vi "FTW-Test-Reflection-Datatypes.vi"() -> (0 "Test Result":errorcluster)   [LabVIEW 2014]
uses:
  src/reflection/FTW-Reflection-Types.ctl
  src/database/core/FTW-SQLite-Core-AccessMode.ctl
  src/socket/inbox/core/FTW-Inbox-Core-Type.ctl
  src/json/core/FTW-JSON-Core-Structure.ctl
  src/error/FTW-ERR-ThrowError.vi
  src/error/FTW-ERR-CallChain.vi
  src/string/FTW-STR-ReplaceWhitespace.vi
panel:
  out "Results Array":T2(array[cluster])
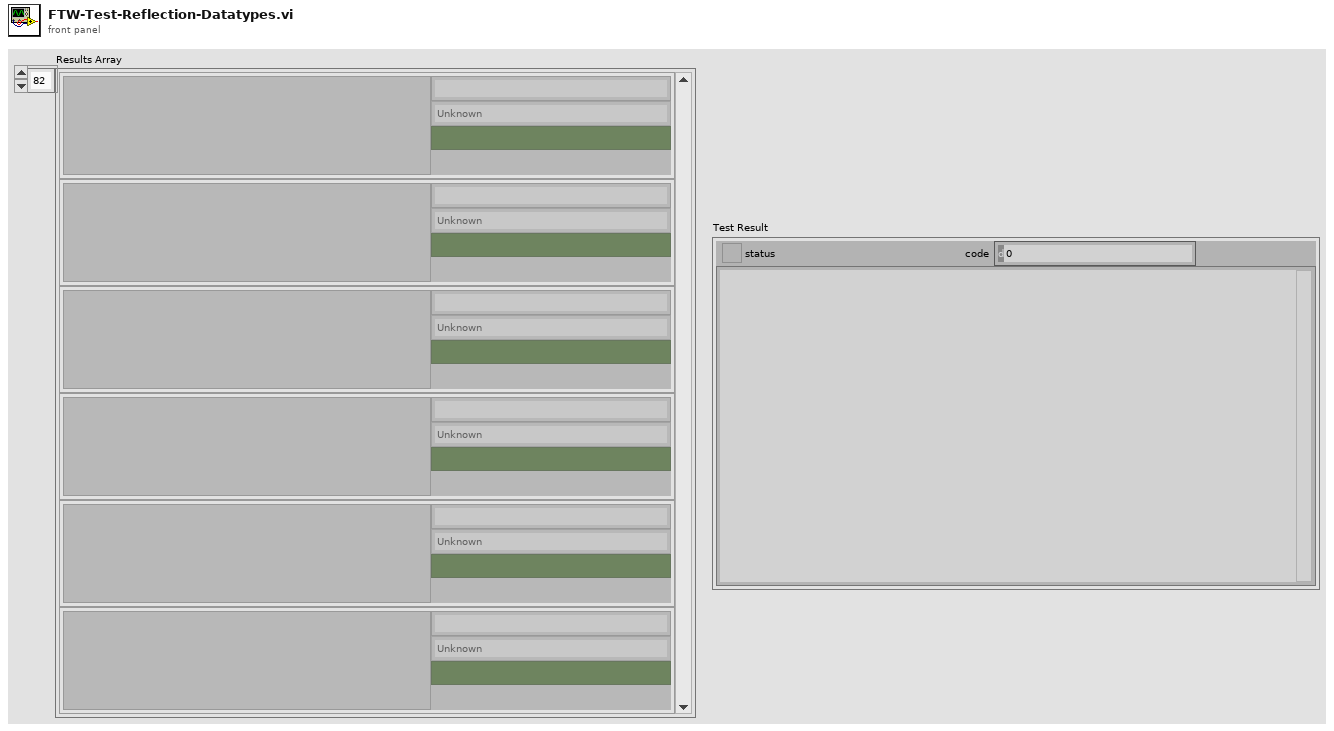
[diagram p1: front panel]
types:
  T1 = typedef "FTW-Reflection-Types.ctl" = enum16{"Unknown", "Void", "Array", "Cluster", "LVObject", "Boolean", "I8", "I16", "I32", "I64", "U8", "U16", "U32", "U64", "SGL", "DBL", "EXT", "CSG", "CDB", "CXT", "FXP", "EnumU8", "EnumU16", "EnumU32", "EnumU64", "SGLwithUnit", "DBLwithUnit", "EXTwithUnit", "CSGwithUnit", "CDBwithUnit", "CXTwithUnit", "String", "Path", "Picture", "Tag", "LVVariant", "Timestamp", "WaveformI8", "WaveformI16", "WaveformI32", "WaveformI64", "WaveformU8", "WaveformU16", "WaveformU32", "WaveformU64", "WaveformSGL", "WaveformDBL", "WaveformEXT", "WaveformCSG", "WaveformCDB", "WaveformCXT", "WaveformDigital", "WaveformUnknownType", "DigitalData", "DynamicData", "ExternalData", "FileByteStream", "TDMStream", "dotNET", "ActiveX", "VIServerReference", "VIReference", "ApplicationInstance", "Menu", "ConnectionDataSocket", "ConnectionVISA", "ConnectionBluetooth", "ConnectionIrDA", "ConnectionTCP", "ConnectionUDP", "ConnectionHTTPClient", "ConnectionFTP", "Occurrence", "Notifier", "Queue", "Rendezvous", "Semaphore", "RTFIFO", "EventPublisher", "EventRegistration", "EventCallback", "DataValueReference", "GenericClass", "GenericClassTag", "GenericClassDeepCopy", "GenericClassFlattened", "GenericClassTagFlattened", "GenericReferenceType", "WindowsRegistry", "OverloadedDatalogRef", "ReferenceUnknownType", "ByteArray", "ConPaneInterface"}
  T2 = cluster{"Variant":variant, "xml string":string, "LabVIEW Type":T1, "Pass?":bool}[]
  T3 = typedef "FTW-Inbox-Core-Type.ctl" = cluster{"Socket":i64, "MessageNotifier":refnum<user-event>, "Message Broker":refnum<user-event>}
  T4 = typedef "Rendezvous RefNum" = refnum<k1>
  T5 = typedef "Semaphore RefNum" = refnum<k1>
  T6 = typedef "FTW-SQLite-Core-AccessMode.ctl" = enum16{"Read", "Read/Write", "Read/Write/Create"}
  T7 = cluster{"Variant":variant, "Match":string, "LabVIEW Type":T1, "Status OK?":bool}
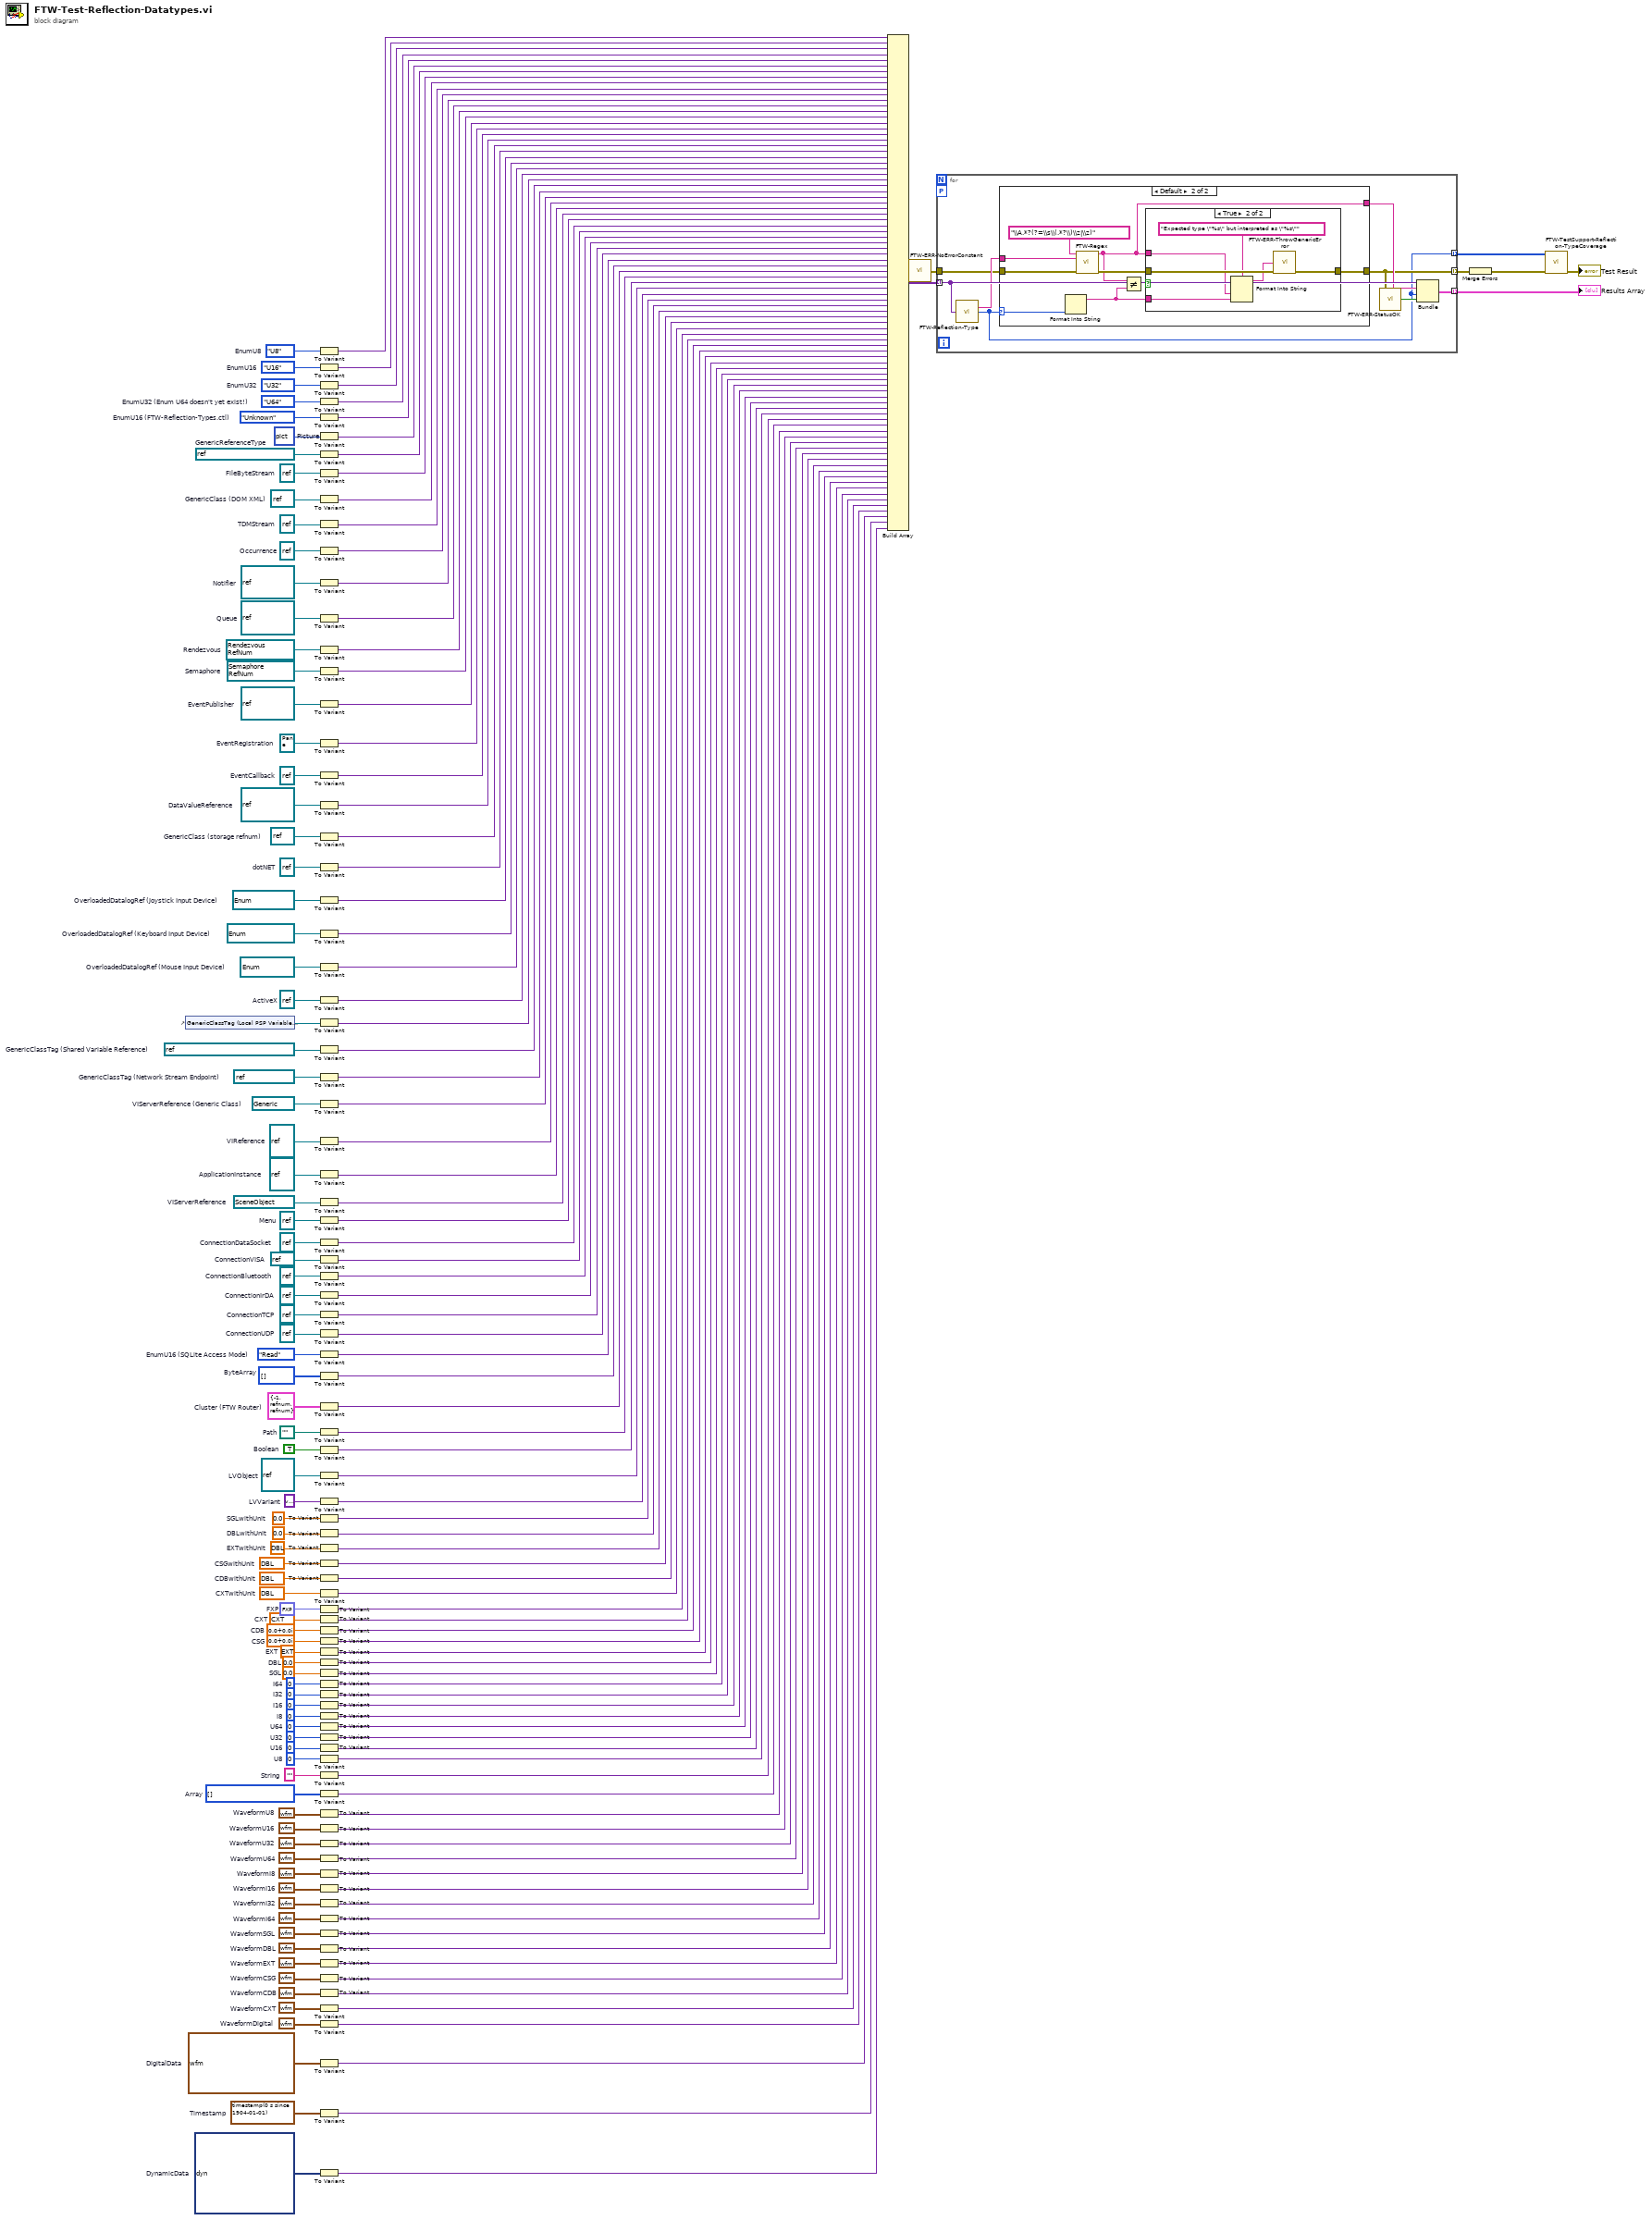
[diagram p0: block diagram]
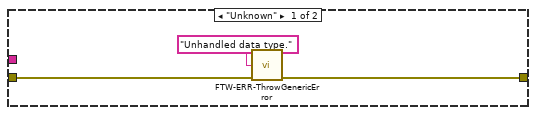
[diagram p2: hidden frame]
diagram:
  w21 = dynamicdata []  # DynamicData
  w5 = u8[] []  # ByteArray
  w6 = T3 {"Socket"=-1, "MessageNotifier"=refnum, "Message Broker"=refnum}  # Cluster (FTW Router)
  w14 = u16[] []  # Array
  w13 = ""  # String
  w9 = T4 refnum items=["rendezvous"]  # Rendezvous
  w8 = T5 refnum items=["semaphore"]  # Semaphore
  w17 = enum32{"U64"}."U64"  # EnumU32 (Enum U64 doesn't yet exist!)
  w20 = FTW-SQLite-Core-AccessMode."Read"  # EnumU16 (SQLite Access Mode)
  w23 = digitalwaveform {"t0"=timestamp(0 s since 1904-01-01), "dt"=0.0, "Y"={"transitions"=[], "data"=[]}}  # WaveformDigital
  w24 = waveform(cxt) {"t0"=timestamp(0 s since 1904-01-01), "dt"=1.0, "Y"=[]}  # WaveformCXT
  w25 = waveform(cdb) {"t0"=timestamp(0 s since 1904-01-01), "dt"=1.0, "Y"=[]}  # WaveformCDB
  w26 = waveform(csg) {"t0"=timestamp(0 s since 1904-01-01), "dt"=1.0, "Y"=[]}  # WaveformCSG
  w27 = waveform(ext) {"t0"=timestamp(0 s since 1904-01-01), "dt"=1.0, "Y"=[]}  # WaveformEXT
  w28 = waveform(dbl) {"t0"=timestamp(0 s since 1904-01-01), "dt"=1.0, "Y"=[]}  # WaveformDBL
  w29 = waveform(sgl) {"t0"=timestamp(0 s since 1904-01-01), "dt"=1.0, "Y"=[]}  # WaveformSGL
  w30 = waveform(i64) {"t0"=timestamp(0 s since 1904-01-01), "dt"=1.0, "Y"=[]}  # WaveformI64
  w31 = waveform(i32) {"t0"=timestamp(0 s since 1904-01-01), "dt"=1.0, "Y"=[]}  # WaveformI32
  w32 = waveform(i16) {"t0"=timestamp(0 s since 1904-01-01), "dt"=1.0, "Y"=[]}  # WaveformI16
  w36 = waveform(i8) {"t0"=timestamp(0 s since 1904-01-01), "dt"=1.0, "Y"=[]}  # WaveformI8
  w37 = waveform(u64) {"t0"=timestamp(0 s since 1904-01-01), "dt"=1.0, "Y"=[]}  # WaveformU64
  w35 = waveform(u32) {"t0"=timestamp(0 s since 1904-01-01), "dt"=1.0, "Y"=[]}  # WaveformU32
  w34 = waveform(u16) {"t0"=timestamp(0 s since 1904-01-01), "dt"=1.0, "Y"=[]}  # WaveformU16
  w33 = waveform(u8) {"t0"=timestamp(0 s since 1904-01-01), "dt"=1.0, "Y"=[]}  # WaveformU8
  w110 = refnum<k31> refnum  # ConnectionBluetooth
  w81 = enum32{"U32"}."U32"  # EnumU32
  w80 = enum16{"U16"}."U16"  # EnumU16
  w79 = enum8{"U8"}."U8"  # EnumU8
  w114 = TRUE  # Boolean
  w115 = path ""  # Path
  w82 = FTW-Reflection-Types."Unknown"  # EnumU16 (FTW-Reflection-Types.ctl)
  w90 = refnum<event-registration> refnum  # EventRegistration
  w113 = refnum<k16> refnum  # ConnectionUDP
  w112 = refnum<k5> refnum  # ConnectionTCP
  w108 = refnum<k13> refnum  # ConnectionDataSocket
  w107 = refnum<k9> refnum  # Menu
  w92 = refnum<data-value> refnum  # DataValueReference
  w111 = refnum<k19> refnum  # ConnectionIrDA
  w83 = picture data[5B]  # Picture
  w106 = refnum<vi> refnum  # VIServerReference
  w104 = refnum<vi> refnum  # ApplicationInstance
  w105 = refnum<vi> refnum  # VIReference
  w103 = refnum<vi> refnum  # VIServerReference (Generic Class)
  w102 = refnum<k21> "localhost"  # GenericClassTag (Network Stream Endpoint)
  w93 = refnum<k27> refnum  # EventCallback
  w91 = refnum<user-event> refnum  # EventPublisher
  w88 = refnum<k4> refnum  # Occurrence
  w10 = refnum<queue> refnum  # Queue
  w89 = refnum<notifier> refnum  # Notifier
  w101 = refnum<k21> "ni.var.psp://localhost/System"  # GenericClassTag (Shared Variable Reference)
  w99 = refnum<k7> refnum  # ActiveX
  w98 = refnum<k1> refnum items=["MOUSE"]  # OverloadedDatalogRef (Mouse Input Device)
  w96 = refnum<k1> refnum items=["KEYBOARD"]  # OverloadedDatalogRef (Keyboard Input Device)
  w97 = refnum<k1> refnum items=["JOYSTICK"]  # OverloadedDatalogRef (Joystick Input Device)
  w94 = refnum<k24> refnum  # dotNET
  w95 = refnum<k20> refnum  # GenericClass (storage refnum)
  w87 = refnum<k34> refnum  # TDMStream
  w84 = refnum<k0> refnum  # GenericReferenceType
  w109 = refnum<visa-resource-name> refnum  # ConnectionVISA
  w86 = refnum<k20> refnum  # GenericClass (DOM XML)
  w85 = refnum<file> refnum  # FileByteStream
  w117 = refnum<class> refnum  # LVObject
  w119 = variant  # LVVariant
  w131 = cxt[unit] 0.0+0.0i  # CXTwithUnit
  w130 = cdb[unit] 0.0+0.0i  # CDBwithUnit
  w129 = csg[unit] 0.0+0.0i  # CSGwithUnit
  w128 = ext[unit] 0.0  # EXTwithUnit
  w127 = dbl[unit] 0.0  # DBLwithUnit
  w126 = sgl[unit] 0.0  # SGLwithUnit
  w178 = timestamp(0 s since 1904-01-01)  # Timestamp
  w148 = cxt 0.0+0.0i  # CXT
  w149 = cdb 0.0+0.0i  # CDB
  w150 = csg 0.0+0.0i  # CSG
  w147 = fxp<+/-,64,1024> 0.0  # FXP
  w151 = ext 0.0  # EXT
  w152 = 0.0  # DBL
  w153 = sgl 0.0  # SGL
  w154 = i64 0  # I64
  w155 = 0  # I32
  w156 = i16 0  # I16
  w157 = i8 0  # I8
  w158 = u64 0  # U64
  w159 = u32 0  # U32
  w160 = u16 0  # U16
  w161 = u8 0  # U8
  w181 = digitaldata {"transitions"=[], "data"=[]}  # DigitalData
  n1 = control-ref of="GenericClassTag (Local PSP Variable Engine)"() -> (w100:refnum<k21>)
  n2 = To Variant(anything=w79) -> (Variant=w7:variant)
  n3 = To Variant(anything=w80) -> (Variant=w39:variant)
  n4 = To Variant(anything=w81) -> (Variant=w15:variant)
  n5 = To Variant(anything=w17) -> (Variant=w16:variant)
  n6 = To Variant(anything=w82) -> (Variant=w40:variant)
  n7 = To Variant(anything=w83) -> (Variant=w41:variant)
  n8 = To Variant(anything=w84) -> (Variant=w42:variant)
  n9 = To Variant(anything=w85) -> (Variant=w43:variant)
  n10 = To Variant(anything=w86) -> (Variant=w44:variant)
  n11 = To Variant(anything=w87) -> (Variant=w45:variant)
  n12 = To Variant(anything=w88) -> (Variant=w46:variant)
  n13 = To Variant(anything=w89) -> (Variant=w47:variant)
  n14 = To Variant(anything=w10) -> (Variant=w48:variant)
  n15 = To Variant(anything=w9) -> (Variant=w49:variant)
  n16 = To Variant(anything=w8) -> (Variant=w50:variant)
  n17 = To Variant(anything=w91) -> (Variant=w51:variant)
  n18 = To Variant(anything=w90) -> (Variant=w52:variant)
  n19 = To Variant(anything=w93) -> (Variant=w53:variant)
  n20 = To Variant(anything=w92) -> (Variant=w54:variant)
  n21 = To Variant(anything=w95) -> (Variant=w55:variant)
  n22 = To Variant(anything=w94) -> (Variant=w56:variant)
  n23 = To Variant(anything=w97) -> (Variant=w57:variant)
  n24 = To Variant(anything=w96) -> (Variant=w58:variant)
  n25 = To Variant(anything=w98) -> (Variant=w59:variant)
  n26 = To Variant(anything=w99) -> (Variant=w60:variant)
  n27 = To Variant(anything=w100) -> (Variant=w61:variant)
  n28 = To Variant(anything=w101) -> (Variant=w62:variant)
  n29 = To Variant(anything=w102) -> (Variant=w63:variant)
  n30 = To Variant(anything=w103) -> (Variant=w64:variant)
  n31 = To Variant(anything=w105) -> (Variant=w65:variant)
  n32 = To Variant(anything=w104) -> (Variant=w66:variant)
  n33 = To Variant(anything=w106) -> (Variant=w67:variant)
  n34 = To Variant(anything=w107) -> (Variant=w68:variant)
  n35 = To Variant(anything=w108) -> (Variant=w69:variant)
  n36 = To Variant(anything=w109) -> (Variant=w70:variant)
  n37 = To Variant(anything=w110) -> (Variant=w71:variant)
  n38 = To Variant(anything=w111) -> (Variant=w72:variant)
  n39 = To Variant(anything=w112) -> (Variant=w73:variant)
  n40 = To Variant(anything=w113) -> (Variant=w74:variant)
  n41 = To Variant(anything=w20) -> (Variant=w75:variant)
  n42 = To Variant(anything=w5) -> (Variant=w4:variant)
  n43 = To Variant(anything=w6) -> (Variant=w76:variant)
  n44 = To Variant(anything=w115) -> (Variant=w77:variant)
  n45 = To Variant(anything=w114) -> (Variant=w78:variant)
  n46 = To Variant(anything=w117) -> (Variant=w116:variant)
  n47 = To Variant(anything=w119) -> (Variant=w118:variant)
  n48 = To Variant(anything=w126) -> (Variant=w120:variant)
  n49 = To Variant(anything=w127) -> (Variant=w121:variant)
  n50 = To Variant(anything=w128) -> (Variant=w122:variant)
  n51 = To Variant(anything=w129) -> (Variant=w123:variant)
  n52 = To Variant(anything=w130) -> (Variant=w124:variant)
  n53 = To Variant(anything=w131) -> (Variant=w125:variant)
  n54 = To Variant(anything=w147) -> (Variant=w132:variant)
  n55 = To Variant(anything=w148) -> (Variant=w133:variant)
  n56 = To Variant(anything=w149) -> (Variant=w134:variant)
  n57 = To Variant(anything=w150) -> (Variant=w135:variant)
  n58 = To Variant(anything=w151) -> (Variant=w136:variant)
  n59 = To Variant(anything=w152) -> (Variant=w137:variant)
  n60 = To Variant(anything=w153) -> (Variant=w138:variant)
  n61 = To Variant(anything=w154) -> (Variant=w139:variant)
  n62 = To Variant(anything=w155) -> (Variant=w140:variant)
  n63 = To Variant(anything=w156) -> (Variant=w141:variant)
  n64 = To Variant(anything=w157) -> (Variant=w142:variant)
  n65 = To Variant(anything=w158) -> (Variant=w143:variant)
  n66 = To Variant(anything=w159) -> (Variant=w144:variant)
  n67 = To Variant(anything=w160) -> (Variant=w145:variant)
  n68 = To Variant(anything=w161) -> (Variant=w146:variant)
  n69 = To Variant(anything=w13) -> (Variant=w12:variant)
  n70 = To Variant(anything=w14) -> (Variant=w11:variant)
  n71 = To Variant(anything=w33) -> (Variant=w177:variant)
  n72 = To Variant(anything=w34) -> (Variant=w176:variant)
  n73 = To Variant(anything=w35) -> (Variant=w175:variant)
  n74 = To Variant(anything=w37) -> (Variant=w174:variant)
  n75 = To Variant(anything=w36) -> (Variant=w173:variant)
  n76 = To Variant(anything=w32) -> (Variant=w172:variant)
  n77 = To Variant(anything=w31) -> (Variant=w171:variant)
  n78 = To Variant(anything=w30) -> (Variant=w170:variant)
  n79 = To Variant(anything=w29) -> (Variant=w169:variant)
  n80 = To Variant(anything=w28) -> (Variant=w168:variant)
  n81 = To Variant(anything=w27) -> (Variant=w167:variant)
  n82 = To Variant(anything=w26) -> (Variant=w166:variant)
  n83 = To Variant(anything=w25) -> (Variant=w165:variant)
  n84 = To Variant(anything=w24) -> (Variant=w164:variant)
  n85 = To Variant(anything=w23) -> (Variant=w163:variant)
  n86 = To Variant(anything=w181) -> (Variant=w162:variant)
  n87 = To Variant(anything=w178) -> (Variant=w38:variant)
  n88 = To Variant(anything=w21) -> (Variant=w22:variant)
  n89 = Build Array(w7, w39, w15, w16, w40, w41, w42, w43, w44, w45, w46, w47, w48, w49, w50, w51, w52, w53, w54, w55, w56, w57, w58, w59, w60, w61, w62, w63, w64, w65, w66, w67, w68, w69, w70, w71, w72, w73, w74, w75, w4, w76, w77, w78, w116, w118, w120, w121, w122, w123, w124, w125, w132, w133, w134, w135, w136, w137, w138, w139, w140, w141, w142, w143, w144, w145, w146, w12, w11, w177, w176, w175, w174, w173, w172, w171, w170, w169, w168, w167, w166, w165, w164, w163, w162, w38, w22) -> (w179:variant[])
  n90 = call "FTW-ERR-NoErrorConstant.vi"() -> ("no error"=w19:errorcluster)
  n91 = for {
    tunnel: w179 -> [w188] mode=indexing
    tunnel: [w189] -> w180 mode=indexing
    tunnel: w19 -> [w186]
    workers-P: _ -> [_]
    tunnel: [w184] -> w18 mode=indexing
    tunnel: [w182] -> w1 mode=indexing
    n92 = call "FTW-Reflection-Type.vi"("Anything"=w188) -> ("Data Name"=w187:string, "LabVIEW Type"=w182:T1)  [unwired: 12 in, 1 out]
    n93 = case shown="Default" w182 {
      selector: w182 -> [_ w198]
      tunnel: w187 -> [_ w201]
      tunnel: w186 -> [w191 w200]
      tunnel: [w190 w195] -> w184
      tunnel: [_ w193] -> w185
      frame "Unknown" {
        n94 = call "FTW-ERR-ThrowGenericError.vi"("Error Message"="Unhandled data type.", "error in"=w191) -> ("error out"=w190:errorcluster)  [unwired: 13 in]
      }
      frame Default {
        n95 = Format Into String(w198) -> (resulting string=w194:string)  [unwired: 3 in, 1 out]
        n96 = call "FTW-Regex.vi"("Regular Expression"="\\A.*?(?=\\s\\(.*?\\)\\z|\\z)", "Input String"=w201, "error in"=w200) -> ("Match"=w193:string, "error out"=w196:errorcluster)  [unwired: 8 in, 3 out]
        n97 = Not Equal?(x=w193, y=w194) -> (x != y?=w197:bool)
        n98 = case shown="True" w197 {
          tunnel: w196 -> [w202 w208]
          tunnel: [w202 w207] -> w195
          tunnel: w193 -> [_ w206]
          tunnel: w194 -> [_ w205]
          frame False {
          }
          frame True {
            n99 = Format Into String(format string="Expected type \"%s\" but interpreted as \"%s\"", w206, w205) -> (resulting string=w203:string)  [unwired: 2 in, 1 out]
            n100 = call "FTW-ERR-ThrowGenericError.vi"("Error Message"=w203, "error in"=w208) -> ("error out"=w207:errorcluster)  [unwired: 13 in]
          }
        }
      }
    }
    n101 = call "FTW-ERR-StatusOK.vi"("error to check"=w184) -> ("Status OK?"=w183:bool)
    n102 = Bundle("Variant"=w188, "Match"=w185, "LabVIEW Type"=w182, "Status OK?"=w183) -> (w189:T7)  [unwired: 1 in]
  }
  "Results Array" <- w180
  n103 = Merge Errors(w18) -> (w3:errorcluster)
  n104 = call "FTW-TestSupport-Reflection-TypeCoverage.vi"("Types Tested"=w1, "error in"=w3) -> ("error out"=→"Test Result":errorcluster)  [unwired: 13 in]
